vi "相机1拍照.vi"(8 "错误输入":errorcluster caption="错误输入（无错误）", 9 "切换曝光时间用Snap？":bool=TRUE, 10 "Image":T2, 11 "引用句柄输入":T1) -> (0 "错误输出":errorcluster, 1 "拍照结果":bool, 2 "Image Out":T2, 3 "引用句柄输出":T1, 4 "取像时间":u32)   [LabVIEW 2014]
uses:
  <vilib>/vision/Image Controls.llb/IMAQ Image.ctl
  <vilib>/userdefined/High Color/IMAQdx.ctl
  <vilib>/vision/driver/NI_Vision_Acquisition_Software.lvlib
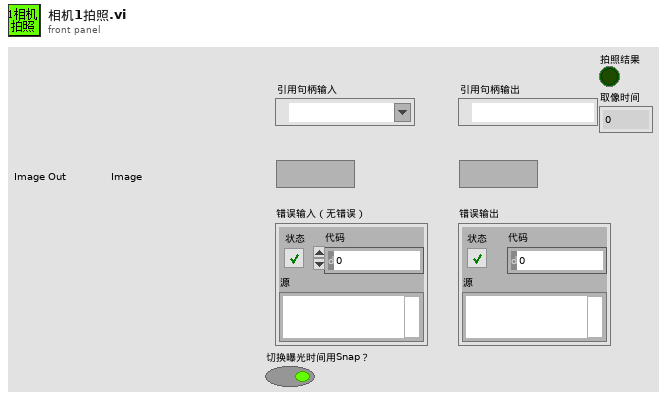
[diagram p1: front panel]
types:
  T1 = typedef "IMAQdx.ctl" = refnum<k21>
  T2 = typedef "IMAQ Image.ctl" = refnum<image>
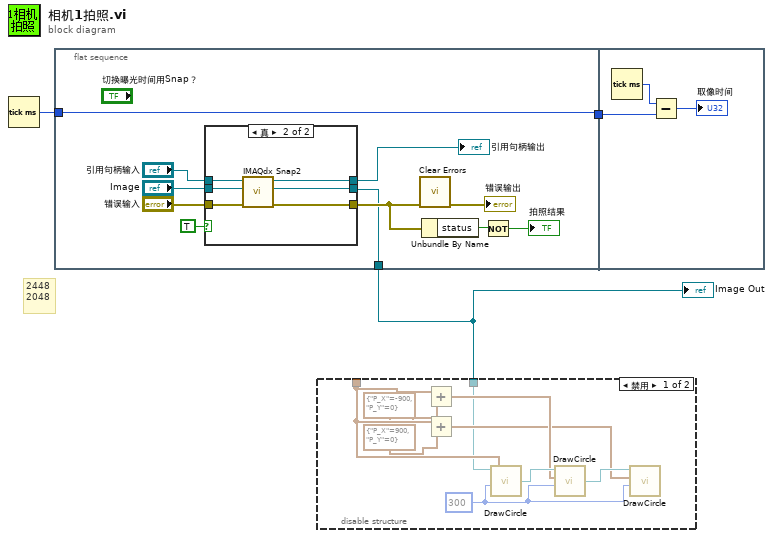
[diagram p0: block diagram]
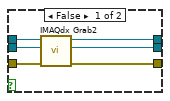
[diagram p3: hidden frame]
diagram:
  # "2448\n2048"
  n1 = Tick Count (ms)() -> (millisecond timer value=w3:u32)
  n2 = flat-sequence {
    tunnel: [w7] -> w1
    tunnel: w3 -> [w6]
    tunnel: [w6] -> w2
    tunnel: w2 -> [w28]
    frame #0 {
      n3 = case shown="真" TRUE {
        tunnel: "Image" -> [w20 w25]
        tunnel: [w19 w23] -> w5
        tunnel: "错误输入" -> [w18 w24]
        tunnel: "引用句柄输入" -> [w17 w26]
        tunnel: [w16 w21] -> w9
        tunnel: [w15 w22] -> w7
        frame False {
          n4 = call <vilib>:"IMAQdx Grab2.vi"("error in"=w18, "Image In"=w20, "Session In"=w17) -> ("error out"=w16:errorcluster, "Image Out"=w15:T2, "Session Out"=w19:T1)  [unwired: 5 in, 1 out]
        }
        frame True {
          n5 = call <vilib>:"IMAQdx Snap2.vi"("error in"=w24, "Image In"=w25, "Session In"=w26) -> ("error out"=w21:errorcluster, "Image Out"=w22:T2, "Session Out"=w23:T1)  [unwired: 6 in]
        }
      }
      "引用句柄输出" <- w5
      n6 = call <vilib>:"Clear Errors.vi"("error in (no error)"=w9) -> ("error out"=→"错误输出":errorcluster)  [unwired: 5 in, 1 out]
      n7 = Unbundle By Name(w9) -> ("status"=w11:bool)
      n8 = Not(x=w11) -> (.not. x?=→"拍照结果":bool)
    }
    frame #1 {
      n9 = Tick Count (ms)() -> (millisecond timer value=w29:u32)
      n10 = Subtract(x=w29, y=w28) -> (x-y=→"取像时间":u32)
    }
  }
  n11 = disable-structure shown="禁用" {
    disable-tunnel: _ -> [w35 _]
    disable-tunnel: w1 -> [w30 _]
    frame Disabled {
      w38 = 300 ("Circle_D")
      n12 = Add(x=w35, y=cluster{"P_X":i32, "P_Y":i32} {"P_X"=-900, "P_Y"=0}) -> (x+y=w34:cluster{"P_X":i32, "P_Y":i32})
      n13 = Add(x=w35, y=cluster{"P_X":i32, "P_Y":i32} {"P_X"=900, "P_Y"=0}) -> (x+y=w33:cluster{"P_X":i32, "P_Y":i32})
      n14 = call "DrawCircle.vi"("Circle_D"=w38, "CircleCenterPosition"=w35, "Img in"=w30) -> ("Img out"=w37:T2)  [unwired: 1 in]
      n15 = call "DrawCircle.vi"("Circle_D"=w38, "CircleCenterPosition"=w34, "Img in"=w37) -> ("Img out"=w36:T2)  [unwired: 1 in]
      n16 = call "DrawCircle.vi"("Circle_D"=w38, "CircleCenterPosition"=w33, "Img in"=w36) -> ()  [unwired: 1 in, 1 out]
    }
    frame Enabled {
    }
  }
  "Image Out" <- w1
